vi "Choose_Titles.vi"(1 "Titles to Show":T1[](array[typedef]), 2 "String 3":string, 3 "String 2":string, 4 "String1":string) -> (0 "Title":string)   [LabVIEW 2022 SP3]
uses:
  Choose_Title.ctl
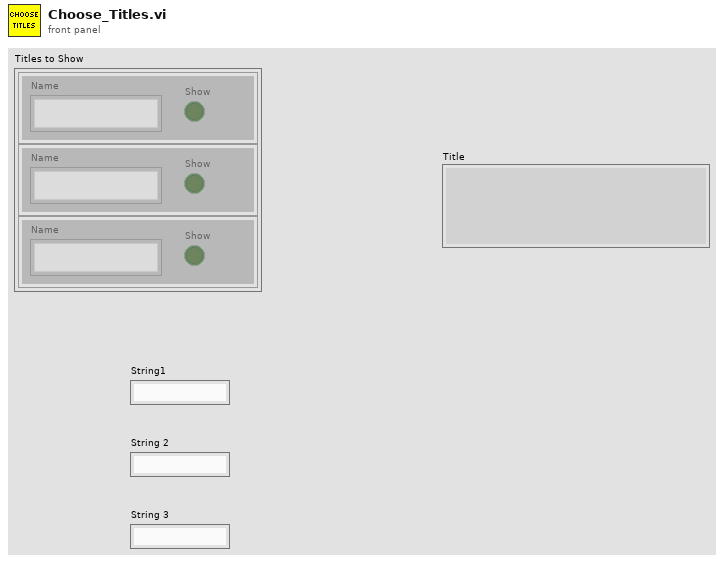
[diagram p1: front panel]
types:
  T1 = typedef "Choose_Title.ctl" = cluster{"Name":string, "Show":bool}
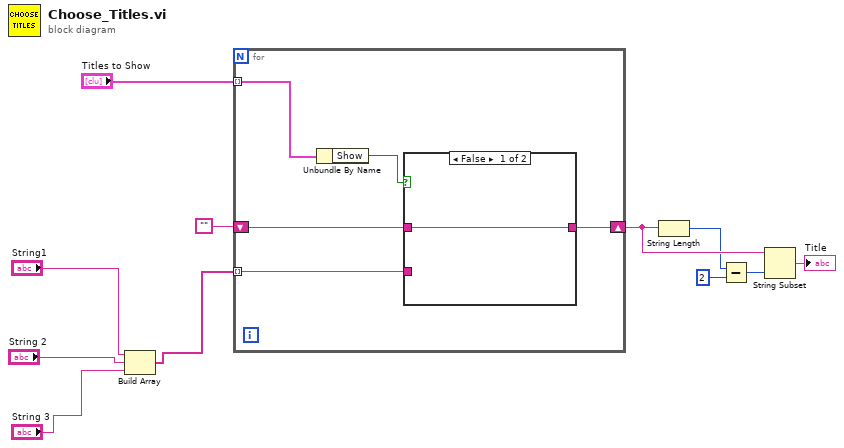
[diagram p0: block diagram]
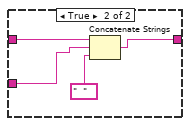
[diagram p2: hidden frame]
diagram:
  n1 = Build Array("String1", "String 2", "String 3") -> (w6:string[])
  n2 = for {
    tunnel: "Titles to Show" -> [w16] mode=indexing
    shift-right: [w12] -> w5
    shift-left: "" -> [w15]
    tunnel: w6 -> [w13] mode=indexing
    n3 = Unbundle By Name(w16) -> ("Show"=w14:bool)
    n4 = case shown="False" w14 {
      tunnel: w15 -> [w17 w21]
      tunnel: w13 -> [_ w20]
      tunnel: [w17 w18] -> w12
      frame False {
      }
      frame True {
        n5 = Concatenate Strings(w21, w20, "  " ("Replace match with:")) -> (w18:string)
      }
    }
  }
  n6 = String Length(string=w5) -> (length=w3:i32)
  n7 = Subtract(x=w3, y=2) -> (x-y=w4:i32)
  n8 = String Subset(string=w5, length (rest)=w4) -> (substring=→"Title":string)  [unwired: 1 in]
